vi "Meas Write Correction Data.vi"(7 "corrections":T1 {"transducers"."channels"."Phase index" min=1 step=1}, 8 "error in":errorcluster, 11 "sequence item":T4) -> (0 "error out":errorcluster)   [LabVIEW 2020]
doc: "Writes loaded correction data into the folder of the new measurement."
uses:
  Meas Sequence Item.ctl
  Meas Sampling Configuration.ctl
  adc/ADC Trig Config.ctl
  adc/ADC Trig Mode Source.ctl
  adc/ADC Trig Slope.ctl
  adc/ADC Trig Coupling.ctl
  processing/QWTB/Meas Proc QWTB Algorithm Parameter Data.ctl
  drivers/DMM/3458A Sampling Rate.ctl
  drivers/AWG/AWG Clock Setup Mode.ctl
  Corrections/Corr Setup.ctl
  Corrections/Corr Tranducer Item.ctl
  Corrections/Corr Digitizers.ctl
  drivers/AWG/AWG.lvlib
  drivers/DMM/3458A Virtual Digitizer.lvlib
panel:
  # "ADC:"
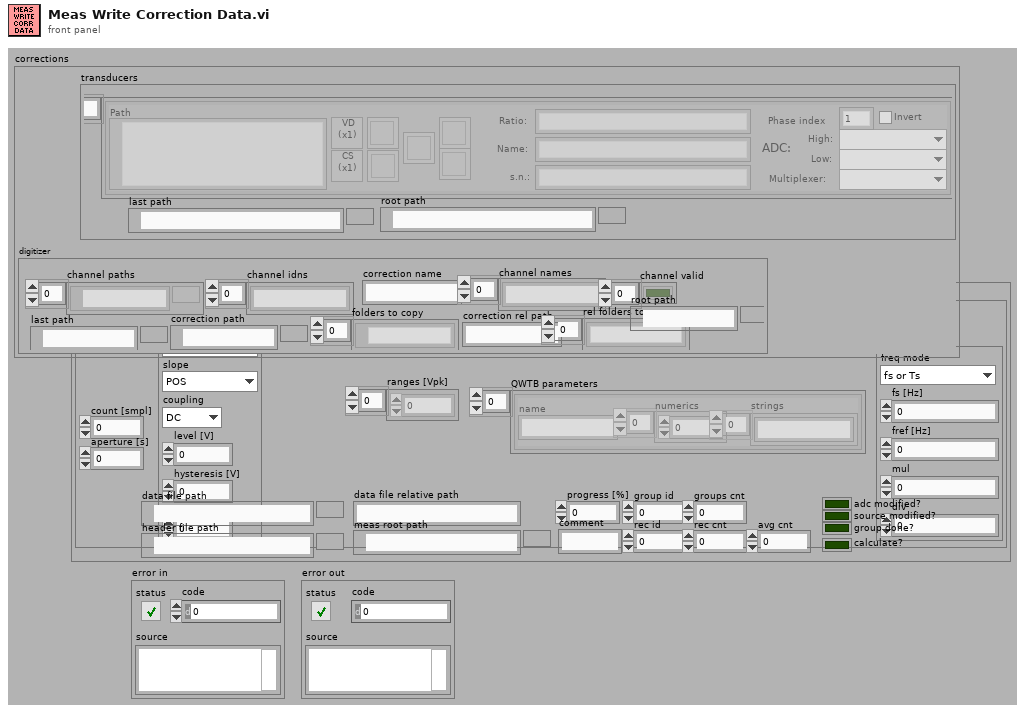
[diagram p1: front panel]
types:
  T1 = typedef "Corr Setup.ctl" = cluster{"transducers":cluster{"channels":T2[], "last path":path, "root path":path}, "digitizer":T3}
  T2 = typedef "Corr Tranducer Item.ctl" = cluster{"Path":path, "Ratio:":string, "Name:":string, "btn rem":bool, "btn up":bool, "btn down":bool, "s.n.:":string, "btn open":bool, "ratio o/i":dbl, "chn hi":u16, "chn lo":u16, "Phase index":i32, "btn edit":bool, "mpx chn":u16, "btn vdx1":bool, "btn csx1":bool, "invert":bool}
  T3 = typedef "Corr Digitizers.ctl" = cluster{"last path":path, "channel paths":path[], "channel idns":string[], "correction name":string, "channel names":string[], "folders to copy":path[], "channel valid":bool[], "correction path":path, "correction rel path":string, "rel folders to copy":string[], "root path":path}
  T4 = typedef "Meas Sequence Item.ctl" = cluster{"config":T5, "data file path":path, "header file path":path, "group id":i32, "rec id":i32, "group done?":bool, "adc modified?":bool, "source modified?":bool, "progress [%]":dbl, "groups cnt":i32, "rec cnt":i32, "data file relative path":string, "meas root path":path, "calculate?":bool, "comment":string, "avg cnt":i32}
  T5 = typedef "Meas Sampling Configuration.ctl" = cluster{"count [smpl]":i64, "aperture [s]":dbl, "trigger":T6, "ranges [Vpk]":dbl[], "QWTB parameters":T10[], "sampling rate":T11}
  T6 = typedef "ADC Trig Config.ctl" = cluster{"source":T7, "slope":T8, "coupling":T9, "level [V]":dbl, "hysteresis [V]":dbl, "pre-trigger [%]":dbl}
  T7 = typedef "ADC Trig Mode Source.ctl" = enum16{"Immediate", "External", "Level"}
  T8 = typedef "ADC Trig Slope.ctl" = enum16{"POS", "NEG"}
  T9 = typedef "ADC Trig Coupling.ctl" = enum16{"DC", "AC"}
  T10 = typedef "Meas Proc QWTB Algorithm Parameter Data.ctl" = cluster{"name":string, "numerics":dbl[], "strings":string[]}
  T11 = typedef "3458A Virtual Digitizer.lvlib/3458A Sampling Rate.ctl" = cluster{"freq mode":T12, "fs [Hz]":dbl, "fref [Hz]":dbl, "mul":dbl, "div":dbl}
  T12 = typedef "AWG.lvlib/AWG Clock Setup Mode.ctl" = enum16{"fs or Ts", "fs or Ts with fref", "fref/N", "fref*M/N", "fref*Ratio"}
  T13 = cluster{"channels":T2[], "last path":path, "root path":path}
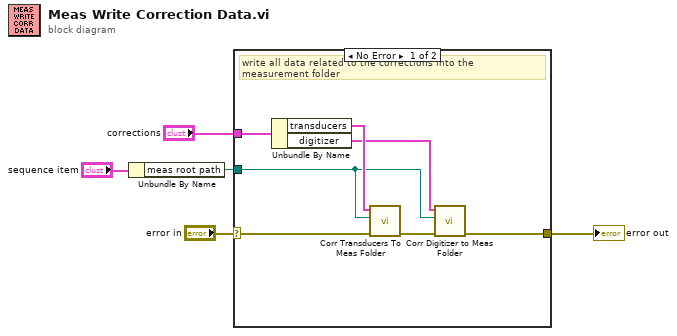
[diagram p0: block diagram]
diagram:
  n1 = Unbundle By Name("sequence item") -> ("meas root path"=w2:path)
  n2 = case shown="No Error" "error in" {
    selector: "error in" -> [w12 w13]
    tunnel: w2 -> [w6 _]
    tunnel: [w8 w13] -> w5
    tunnel: "corrections" -> [w11 _]
    frame No Error {
      # "write all data related to the corrections into the measurement folder"
      n3 = Unbundle By Name(w11) -> ("transducers"=w10:T13, "digitizer"=w7:T3)
      n4 = call "Corr Transducers To Meas Folder.vi"("error in"=w12, "measurement root path"=w6, "transducers in"=w10) -> ("error out"=w9:errorcluster)  [unwired: 7 in, 1 out]
      n5 = call "Corr Digitizer to Meas Folder.vi"("error in"=w9, "measurement root path"=w6, "digitizer corr in"=w7) -> ("error out"=w8:errorcluster)  [unwired: 7 in, 1 out]
    }
    frame Error {
    }
  }
  "error out" <- w5
